vi "Write volume table.vi"(8 "error in (no error)":errorcluster, 9 "File name":path, 10 "Volume map":dbl[][](array[numeric]), 11 "Tomo in":refnum<class "Tomo.lvclass">) -> (0 "error out":errorcluster, 3 "Tomo out":refnum<class "Tomo.lvclass">)   [LabVIEW 2012, in "Tomo.lvclass"]
uses:
  Tomo.lvclass
  <vilib>/Utility/file.llb/Write To Spreadsheet File (DBL).vi
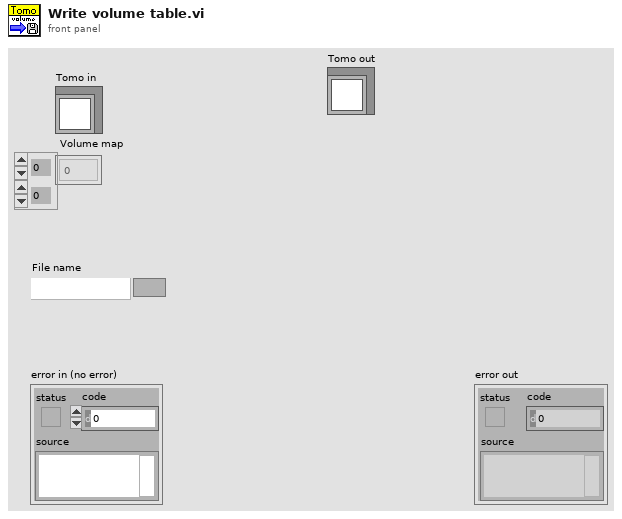
[diagram p1: front panel]
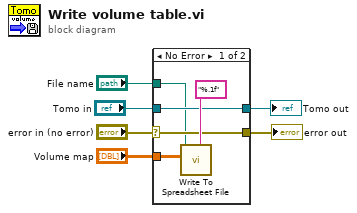
[diagram p0: block diagram]
diagram:
  n1 = case shown="No Error" "error in (no error)" {
    selector: "error in (no error)" -> [w8 w13]
    tunnel: [w8 w13] -> w5
    tunnel: [w9 w12] -> w1
    tunnel: "Tomo in" -> [w9 w12]
    tunnel: "Volume map" -> [w11 _]
    tunnel: "File name" -> [w7 _]
    frame No Error {
      n2 = call-poly <vilib>:"Write To Spreadsheet File.vi"("format (%.3f)"="%.1f", "2D data"=w11, "file path (dialog if empty)"=w7) -> ()  [unwired: 5 in, 1 out]
    }
    frame Error {
    }
  }
  "error out" <- w5
  "Tomo out" <- w1
